vi "Set-Get power set.vi"(8 "error in (no error)":errorcluster, 11 "Input set":i32[](array[numeric])=[2, 3, 7, 11, 17]) -> (0 "error out":errorcluster, 3 "Power set-each variant contains a subset":variant[](array[variant]))   [LabVIEW 2021, in "Numeric Utilities.lvlib"]
uses:
  Numeric Utilities.lvlib
panel:
  out "index of last element":i32
  out "L = desired subset length":i32
  out "Power set-actual no. of elements":u64
  out "Power set-expected no. of elements":u64
  # "Development\ncontrols/indicators useful for development and testing, but which are not outputs of the VI"
  # "Input\nInputs to the VI"
  # "Output\nOutputs of the VI"
  # "Description\n\nBlank VI with error handling case. \n\nSummarize the use of this VI in this space."
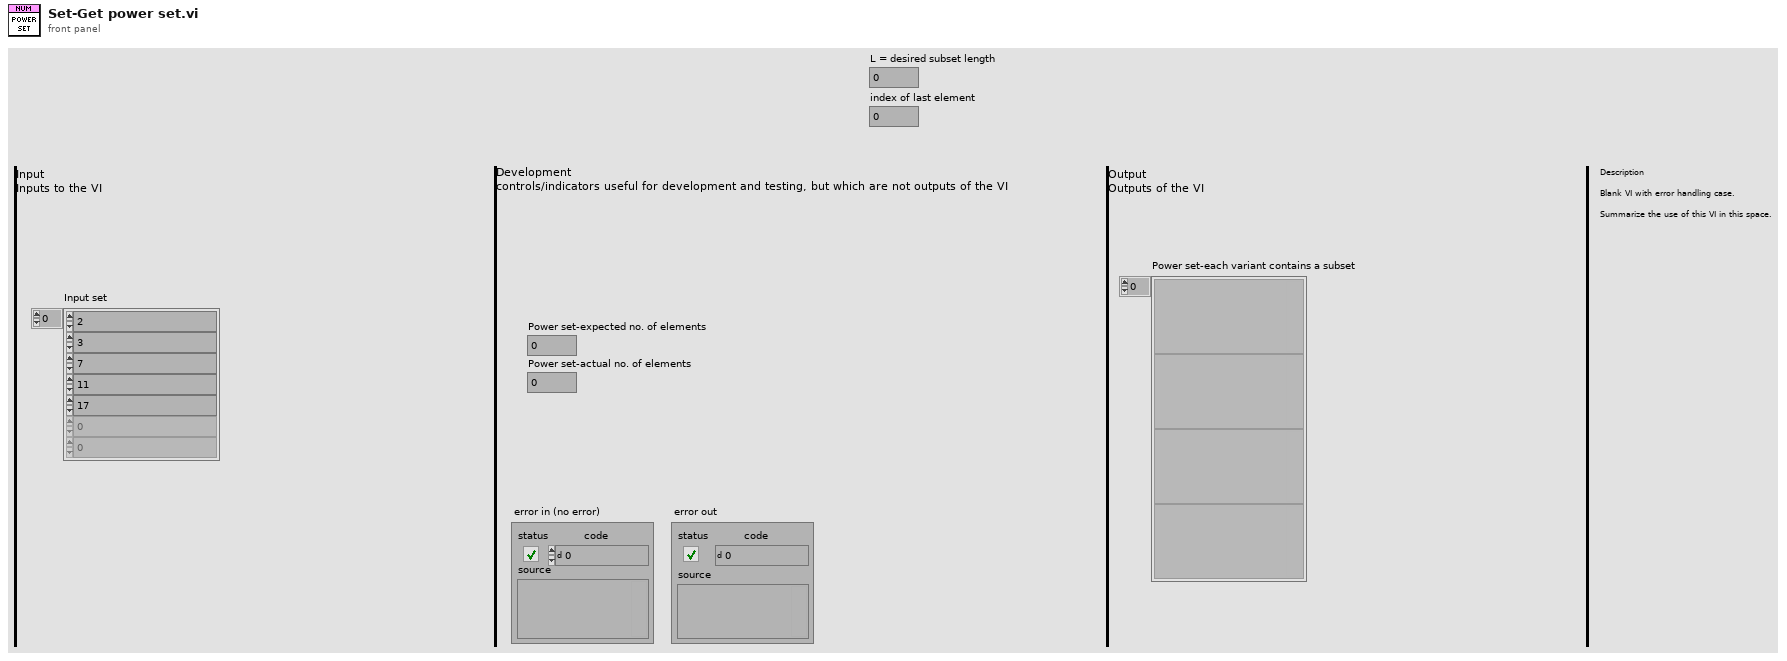
[diagram p1: front panel]
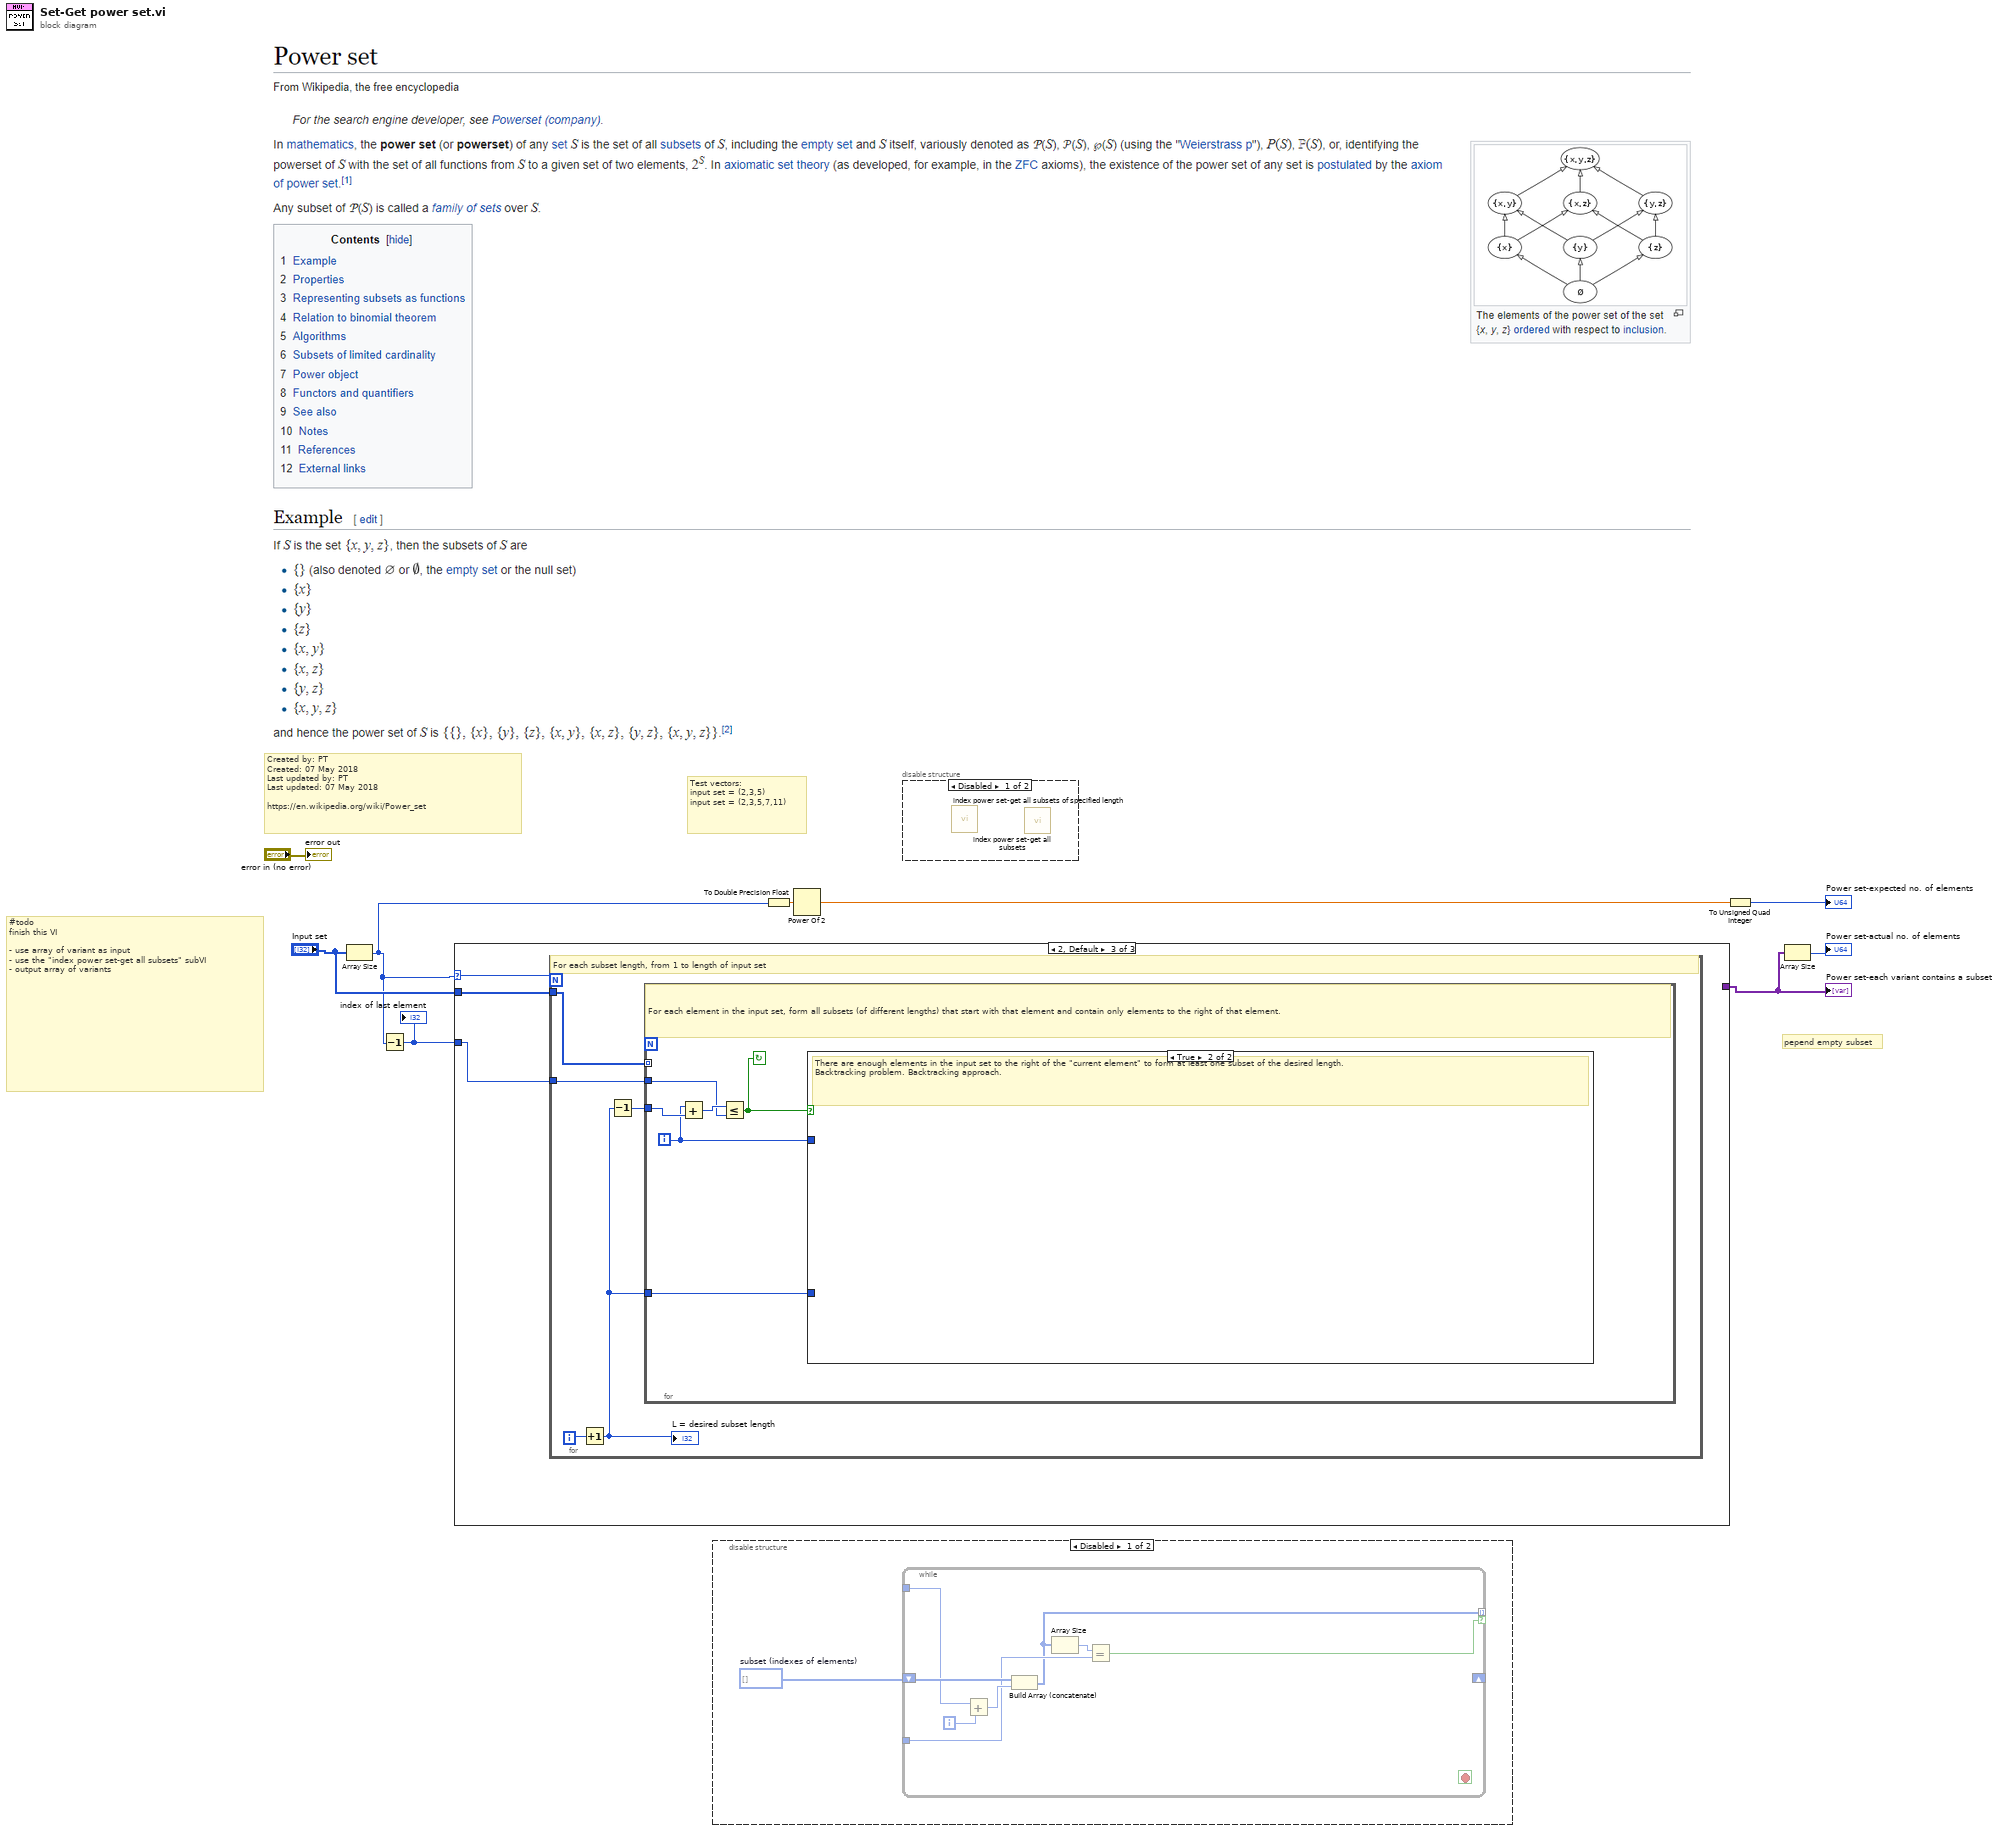
[diagram p0: block diagram]
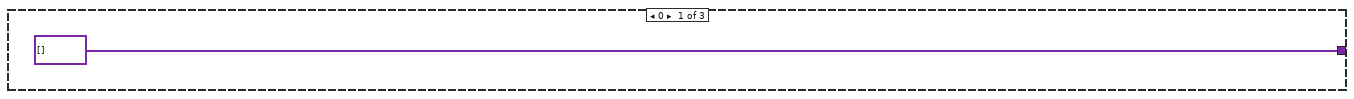
[diagram p4: hidden frame]
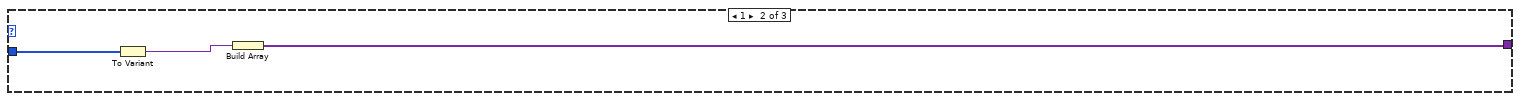
[diagram p5: hidden frame]
diagram:
  # "#todo\nfinish this VI\n\n- use array of variant as input\n- use the \"index power set-get all subsets\" subVI\n- output array of variants"
  # "Test vectors:\ninput set = (2,3,5)\ninput set = (2,3,5,7,11)"
  # "pepend empty subset"
  # "Created by: PT\nCreated: 07 May 2018\nLast updated by: PT\nLast updated: 07 May 2018\n\nhttps://en.wikipedia.org/wiki/Power_set"
  n1 = Array Size(array="Input set") -> (size(s)=w2:i32)
  n2 = Decrement(x=w2) -> (x-1=w1:i32)
  "index of last element" <- w1
  n3 = case shown="2, Default" w2 {
    selector: w2 -> [_ _ w15]
    tunnel: [variant[] [] ("Power set-each variant contains a subset") w11 _] -> w4
    tunnel: "Input set" -> [_ w13 w16]
    tunnel: w1 -> [_ _ w14]
    frame 0 {
    }
    frame 1 {
      n4 = To Variant(anything=w13) -> (Variant=w12:variant)
      n5 = Build Array(w12) -> (w11:variant[])
    }
    frame 2, Default {
      n6 = for {
        N: w15 -> [_]
        tunnel: w16 -> [w20]
        tunnel: w14 -> [w19]
        i -> [w21]
        # "For each subset length, from 1 to length of input set"
        n7 = Increment(x=w21) -> (x+1=w17:i32)
        "L = desired subset length" <- w17
        n8 = Decrement(x=w17) -> (x-1=w18:i32)
        n9 = for {
          tunnel: w20 -> [_] mode=indexing
          tunnel: w18 -> [w27]
          tunnel: w19 -> [w25]
          tunnel: w17 -> [w22]
          i -> [w23]
          stop <- w24 continue-if-true
          # "For each element in the input set, form all subsets (of different lengths) that start with that element and contain only elements to the right of that element."
          n10 = Add(x=w23, y=w27) -> (x+y=w26:i32)
          n11 = Less Or Equal?(x=w26, y=w25) -> (x <= y?=w24:bool)
          n12 = case shown="True" w24 {
            tunnel: w23 -> [_ _]
            tunnel: w22 -> [_ _]
            frame False {
              # "There aren't enough elements left to the right of the \"current element\" to form a subset of the desired length."
            }
            frame True {
              # "There are enough elements in the input set to the right of the \"current element\" to form at least one subset of the desired length.\nBacktracking problem. Backtracking approach."
            }
          }
        }
      }
    }
  }
  "Power set-each variant contains a subset" <- w4
  n13 = disable-structure shown="Disabled" {
    frame Disabled {
      w28 = i32[] []  # subset (indexes of elements)
      n14 = while {
        tunnel: _ -> [w34]
        shift-right: _ -> [_]
        shift-left: w28 -> [w36]
        tunnel: _ -> [w31]
        tunnel: [w30] -> _ mode=indexing if=w29
        i -> [w33]
        stop <- _ stop-if-true
        n15 = Add(x=w34, y=w33) -> (x+y=w35:i32)
        n16 = Build Array (concatenate)(w36, w35) -> (w30:i32[])
        n17 = Array Size(array=w30) -> (size(s)=w32:i32)
        n18 = Equal?(x=w32, y=w31) -> (x = y?=w29:bool)
      }
    }
    frame Enabled {
    }
  }
  n19 = To Double Precision Float(number=w2) -> (double precision float=w8:dbl)
  n20 = Power Of 2(x=w8) -> (2^x=w7:dbl)
  n21 = disable-structure shown="Disabled" {
    frame Disabled {
      n22 = call "index power set-get all subsets of specified length.vi"() -> ()  [unwired: 9 in, 3 out]
      n23 = call "index power set-get all subsets.vi"() -> ()  [unwired: 8 in, 4 out]
    }
    frame Enabled {
    }
  }
  n24 = To Unsigned Quad Integer(1:w7) -> (0:→"Power set-expected no. of elements":u64)
  n25 = Array Size(array=w4) -> (size(s)=→"Power set-actual no. of elements":i32)
  "error out" <- "error in (no error)"
